vi "VL53L0X_DataInit.vi"(11 "REV2mDistanceSensorDevRef":T1) -> (3 "REV2mDistanceSensorDevRef Out":T1)   [LabVIEW 2019, in "DistanceSensorDriver.lvlib"]
uses:
  DistanceSensorDriver.lvlib
  Typedef/REV2mDistanceSensorDevRef.ctl
  Typedef/Ports.ctl
panel:
  out "Port":i32
  out "Address":i32
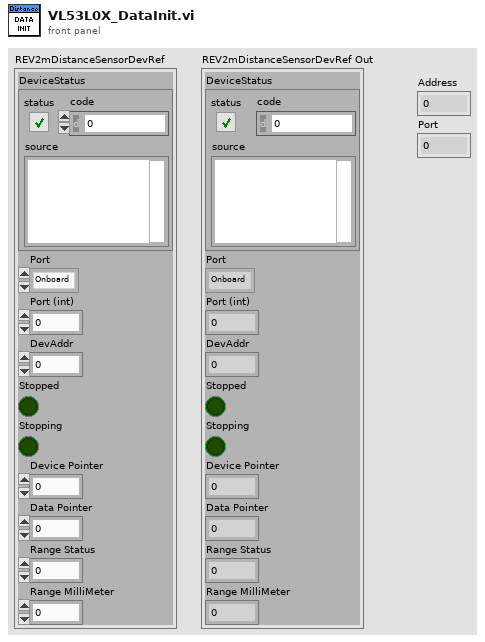
[diagram p1: front panel]
types:
  T1 = typedef "DistanceSensorDriver.lvlib/REV2mDistanceSensorDevRef.ctl" = cluster{"DeviceStatus":errorcluster, "Port":T2, "Port (int)":i32, "DevAddr":i32, "Stopped":bool, "Stopping":bool, "Device Pointer":u64, "Data Pointer":u64, "Range Status":u8, "Range MilliMeter":u16}
  T2 = typedef "DistanceSensorDriver.lvlib/Ports.ctl" = enum32{"Onboard", "MXP"}
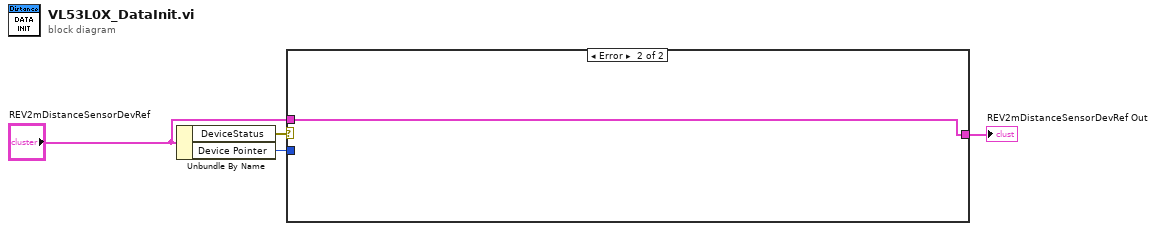
[diagram p0: block diagram]
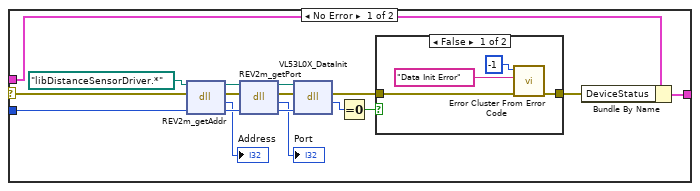
[diagram p2: hidden frame]
diagram:
  n1 = Unbundle By Name("REV2mDistanceSensorDevRef") -> ("DeviceStatus"=w1:errorcluster, "Device Pointer"=w2:u64)
  n2 = case shown="Error" w1 {
    selector: w1 -> [w5 _]
    tunnel: [w17 w27] -> w4
    tunnel: "REV2mDistanceSensorDevRef" -> [w16 w27]
    tunnel: w2 -> [w15 _]
    frame No Error {
      n3 = dll-call lib="?" fn="REV2m_getAddr"(path in=path "libDistanceSensorDriver.*", error in=w5, "Dev"=w15) -> (path out=w11:path, error out=w9:errorcluster, "Address"=→"Address":i32, "Dev"=w14:u64)  [unwired: 1 in]
      n4 = dll-call lib="?" fn="REV2m_getPort"(path in=w11, error in=w9, "Dev"=w14) -> (path out=w10:path, error out=w8:errorcluster, "Port"=→"Port":i32, "Dev"=w13:u64)  [unwired: 1 in]
      n5 = dll-call lib="?" fn="VL53L0X_DataInit"(path in=w10, error in=w8, "Dev"=w13) -> (error out=w18:errorcluster, "Status"=w19:i32)  [unwired: 2 in, 1 out]
      n6 = Equal To 0?(x=w19) -> (x = 0?=w21:bool)
      n7 = case shown="False" w21 {
        tunnel: w18 -> [w22 w26]
        tunnel: [w25 w26] -> w20
        frame False {
          n8 = call <vilib>:"Error Cluster From Error Code.vi"("error in (no error)"=w22, "error message (\"\")"="Data Init Error" ("error message (\"\")"), "error code (0)"=-1) -> ("error out"=w25:errorcluster)  [unwired: 6 in]
        }
        frame True {
        }
      }
      n9 = Bundle By Name(cluster=w16, "DeviceStatus"=w20) -> (w17:T1)
    }
    frame Error {
    }
  }
  "REV2mDistanceSensorDevRef Out" <- w4
